vi "p5.0.vi"() -> ()   [LabVIEW 2020]
uses:
  <vilib>/Analysis/4window.llb/windowTd.ctl
  <vilib>/Analysis/NI_AALPro.lvlib
panel:
  out "DFT dB":dynamicdata(graph)
  out "DFT":dynamicdata(graph)
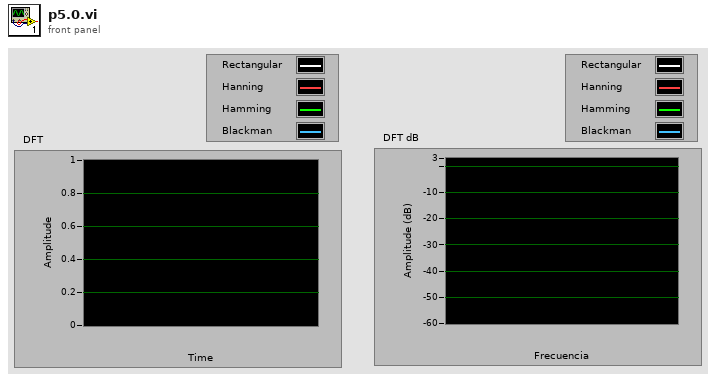
[diagram p1: front panel]
types:
  T1 = typedef "NI_AALPro.lvlib/windowTd.ctl" = u32
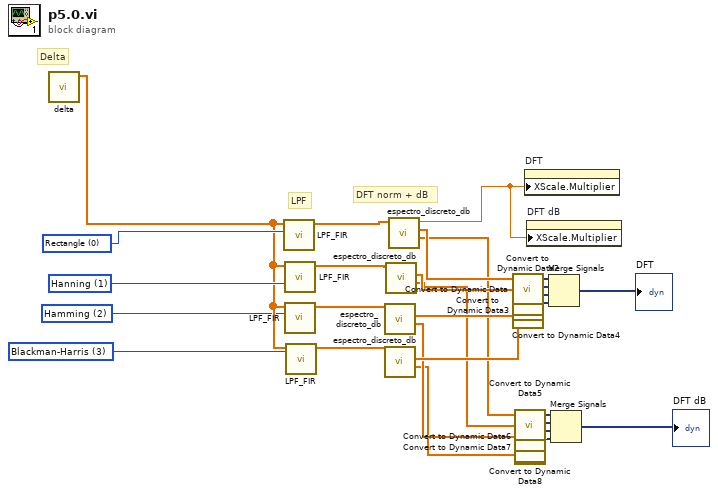
[diagram p0: block diagram]
diagram:
  w23 = T1 3 items=["Rectangle"=0, "Hanning"=1, "Hamming"=2, "Blackman-Harris"=3, "Exact Blackman"=4, "Blackman"=5, "Flat Top"=6, "4 Term B-Harris "=7, "7 Term B-Harris"=8, "Low Sidelobe"=9, "Blackman Nuttall"=11, "Triangle"=30, "Bartlett-Hanning"=31, "Bohman"=32, "Parzen"=33, "Welch"=34, "Kaiser"=60, "Dolph-Chebyshev"=61, "Gaussian"=62] ("window")
  w24 = T1 2 items=["Rectangle"=0, "Hanning"=1, "Hamming"=2, "Blackman-Harris"=3, "Exact Blackman"=4, "Blackman"=5, "Flat Top"=6, "4 Term B-Harris "=7, "7 Term B-Harris"=8, "Low Sidelobe"=9, "Blackman Nuttall"=11, "Triangle"=30, "Bartlett-Hanning"=31, "Bohman"=32, "Parzen"=33, "Welch"=34, "Kaiser"=60, "Dolph-Chebyshev"=61, "Gaussian"=62] ("window")
  w26 = T1 1 items=["Rectangle"=0, "Hanning"=1, "Hamming"=2, "Blackman-Harris"=3, "Exact Blackman"=4, "Blackman"=5, "Flat Top"=6, "4 Term B-Harris "=7, "7 Term B-Harris"=8, "Low Sidelobe"=9, "Blackman Nuttall"=11, "Triangle"=30, "Bartlett-Hanning"=31, "Bohman"=32, "Parzen"=33, "Welch"=34, "Kaiser"=60, "Dolph-Chebyshev"=61, "Gaussian"=62] ("window")
  w27 = T1 0 items=["Rectangle"=0, "Hanning"=1, "Hamming"=2, "Blackman-Harris"=3, "Exact Blackman"=4, "Blackman"=5, "Flat Top"=6, "4 Term B-Harris "=7, "7 Term B-Harris"=8, "Low Sidelobe"=9, "Blackman Nuttall"=11, "Triangle"=30, "Bartlett-Hanning"=31, "Bohman"=32, "Parzen"=33, "Welch"=34, "Kaiser"=60, "Dolph-Chebyshev"=61, "Gaussian"=62] ("window")
  # "LPF"
  # "DFT norm + dB"
  # "Delta"
  n1 = call "delta.vi"() -> ("Array"=w25:dbl[])  [unwired: 11 in]
  n2 = call "LPF_FIR.vi"("window"=w27, "Array"=w25) -> ("Filtered X"=w28:dbl[])  [unwired: 9 in]
  n3 = call "LPF_FIR.vi"("window"=w26, "Array"=w25) -> ("Filtered X"=w22:dbl[])  [unwired: 9 in]
  n4 = call "LPF_FIR.vi"("window"=w24, "Array"=w25) -> ("Filtered X"=w21:dbl[])  [unwired: 9 in]
  n5 = call "LPF_FIR.vi"("window"=w23, "Array"=w25) -> ("Filtered X"=w20:dbl[])  [unwired: 9 in]
  n6 = call "espectro_discreto_db.vi"("Filtered X"=w21) -> ("DFT dB"=w7:dbl[], "DFT"=w15:dbl[])  [unwired: 8 in, 1 out]
  n7 = call "espectro_discreto_db.vi"("Filtered X"=w20) -> ("DFT dB"=w5:dbl[], "DFT"=w13:dbl[])  [unwired: 8 in, 1 out]
  n8 = call "espectro_discreto_db.vi"("Filtered X"=w22) -> ("DFT dB"=w9:dbl[], "DFT"=w17:dbl[])  [unwired: 8 in, 1 out]
  n9 = call "espectro_discreto_db.vi"("Filtered X"=w28) -> ("DFT dB"=w11:dbl[], "DFT"=w19:dbl[], "Multiplier factor"=w1:dbl)  [unwired: 8 in]
  n10 = call "Convert to Dynamic Data"("Array"=w19) -> ("Dynamic Data Type"=w18:dynamicdata)  [unwired: 3 in]
  n11 = call "Convert to Dynamic Data2"("Array"=w17) -> ("Dynamic Data Type"=w16:dynamicdata)  [unwired: 3 in]
  n12 = call "Convert to Dynamic Data3"("Array"=w15) -> ("Dynamic Data Type"=w14:dynamicdata)  [unwired: 3 in]
  n13 = call "Convert to Dynamic Data4"("Array"=w13) -> ("Dynamic Data Type"=w12:dynamicdata)  [unwired: 3 in]
  n14 = call "Convert to Dynamic Data5"("Array"=w11) -> ("Dynamic Data Type"=w10:dynamicdata)  [unwired: 3 in]
  n15 = call "Convert to Dynamic Data6"("Array"=w9) -> ("Dynamic Data Type"=w8:dynamicdata)  [unwired: 3 in]
  n16 = call "Convert to Dynamic Data7"("Array"=w7) -> ("Dynamic Data Type"=w6:dynamicdata)  [unwired: 3 in]
  n17 = call "Convert to Dynamic Data8"("Array"=w5) -> ("Dynamic Data Type"=w4:dynamicdata)  [unwired: 3 in]
  n18 = property on="DFT" class="WFGraph (strict)"("XScale.Multiplier"=w1) -> ()  [unwired: 2 in, 2 out]
  n19 = property on="DFT dB" class="WFGraph (strict)"("XScale.Multiplier"=w1) -> ()  [unwired: 2 in, 2 out]
  n20 = Merge Signals(w18, w16, w14, w12) -> (→"DFT":dynamicdata)
  n21 = Merge Signals(w10, w8, w6, w4) -> (→"DFT dB":dynamicdata)
